vi "添加数据到配置文件.vi"(7 "参数GPRS引用句柄":refnum<vi>, 8 "错误输入（无错误）":errorcluster, 9 "配置文件输入":T1 caption="refnum", 10 "名称":string, 11 "下拉框输入":refnum<vi>) -> (0 "错误输出":errorcluster, 3 "配置文件输出":T1 caption="refnum out")   [LabVIEW 2015]
uses:
  <vilib>/Utility/config.llb/Config Data RefNum.ctl
  <vilib>/Utility/config.llb/Write Key (String).vi
  <vilib>/Utility/config.llb/Write Key (U32).vi
  <vilib>/Utility/config.llb/NI_LVConfig.lvlib
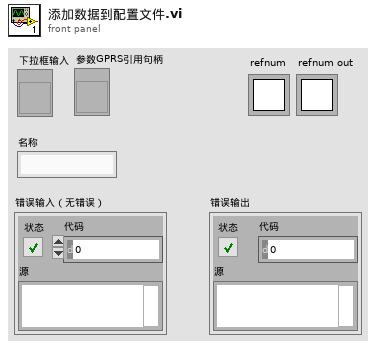
[diagram p1: front panel]
types:
  T1 = typedef "NI_LVConfig.lvlib/Config Data RefNum.ctl" = refnum<k1>
  T2 = typedef "GPRS参数123.ctl" = cluster{"IP地址":string, "端口号":u16, "工作模式":u16, "连接协议":u16, "连接方式":u16, "本机号码":string, "短信监控中心号码1":string, "监听时间":u16, "心跳间隔":u16, "重启时间(分)":u16, "C/S关系":u16, "DNS域名":string, "APN接入点":string, "报头使能":u16, "ID号":string, "波特率":u16, "数据位":u16, "停止位":u16, "校验位":u16, "短信目标号码1 ":string, "短信目标号码2":string, "短信监控中心号码2":string, "信号检测使能":u16, "控制方式":u16}
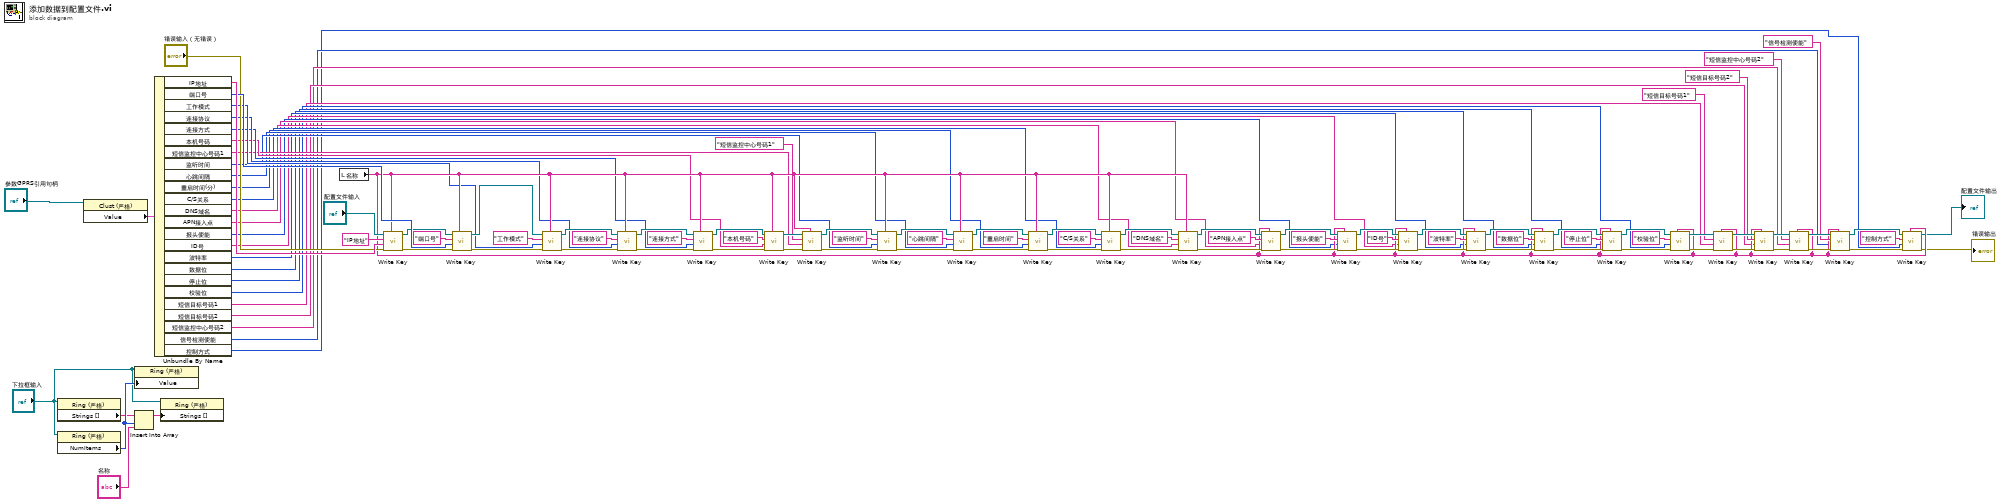
[diagram p0: block diagram]
diagram:
  n1 = property on="属性节点" class="Ring (严格)"(reference="下拉框输入") -> ("Strings []"=w105:string[])  [unwired: 1 in, 2 out]
  n2 = property on="属性节点" class="Ring (严格)"(reference="下拉框输入") -> ("NumItems"=w106:u32)  [unwired: 1 in, 2 out]
  n3 = property class="Clust (严格)"(reference="参数GPRS引用句柄") -> ("Value"=w101:T2)  [unwired: 1 in, 2 out]
  n4 = property on="属性节点" class="Ring (严格)"(reference="下拉框输入", "Value"=w106) -> ()  [unwired: 1 in, 2 out]
  n5 = Insert Into Array(array=w105, index=w106, new element="名称") -> (w104:string[])
  n6 = Unbundle By Name(w101) -> ("IP地址"=w98:string, "端口号"=w96:u16, "工作模式"=w24:u16, "连接协议"=w23:u16, "连接方式"=w22:u16, "本机号码"=w21:string, "短信监控中心号码1"=w20:string, "监听时间"=w19:u16, "心跳间隔"=w18:u16, "重启时间(分)"=w17:u16, "C/S关系"=w16:u16, "DNS域名"=w15:string, "APN接入点"=w14:string, "报头使能"=w13:u16, "ID号"=w12:string, "波特率"=w11:u16, "数据位"=w10:u16, "停止位"=w9:u16, "校验位"=w8:u16, "短信目标号码1"=w7:string, "短信目标号码2"=w6:string, "短信监控中心号码2"=w5:string, "信号检测使能"=w4:u16, "控制方式"=w3:u16)
  n7 = property on="属性节点" class="Ring (严格)"(reference="下拉框输入", "Strings []"=w104) -> ()  [unwired: 1 in, 2 out]
  n8 = local read "名称"() -> (w25:string)
  n9 = call-poly <vilib>:"Write Key.vi"("section"=w25, "error in (no error)"="错误输入（无错误）", "value"=w98, "key"="IP地址", "refnum"="配置文件输入") -> ("error out"=w92:errorcluster, "refnum out"=w94:T1)  [unwired: 4 in, 1 out]
  n10 = call-poly <vilib>:"Write Key.vi"("section"=w25, "error in (no error)"=w92, "value"=w96, "key"="端口号", "refnum"=w94) -> ("error out"=w60:errorcluster, "refnum out"=w61:T1)  [unwired: 4 in, 1 out]
  n11 = call-poly <vilib>:"Write Key.vi"("section"=w25, "error in (no error)"=w60, "value"=w24, "key"="工作模式", "refnum"=w61) -> ("error out"=w91:errorcluster, "refnum out"=w90:T1)  [unwired: 4 in, 1 out]
  n12 = call-poly <vilib>:"Write Key.vi"("section"=w25, "error in (no error)"=w91, "value"=w23, "key"="连接协议", "refnum"=w90) -> ("error out"=w87:errorcluster, "refnum out"=w86:T1)  [unwired: 4 in, 1 out]
  n13 = call-poly <vilib>:"Write Key.vi"("section"=w25, "error in (no error)"=w87, "value"=w22, "key"="连接方式", "refnum"=w86) -> ("error out"=w89:errorcluster, "refnum out"=w88:T1)  [unwired: 4 in, 1 out]
  n14 = call-poly <vilib>:"Write Key.vi"("section"=w25, "error in (no error)"=w89, "value"=w21, "key"="本机号码", "refnum"=w88) -> ("error out"=w79:errorcluster, "refnum out"=w78:T1)  [unwired: 4 in, 1 out]
  n15 = call-poly <vilib>:"Write Key.vi"("section"=w25, "error in (no error)"=w79, "value"=w20, "key"="短信监控中心号码1", "refnum"=w78) -> ("error out"=w85:errorcluster, "refnum out"=w84:T1)  [unwired: 4 in, 1 out]
  n16 = call-poly <vilib>:"Write Key.vi"("section"=w25, "error in (no error)"=w85, "value"=w19, "key"="监听时间", "refnum"=w84) -> ("error out"=w81:errorcluster, "refnum out"=w80:T1)  [unwired: 4 in, 1 out]
  n17 = call-poly <vilib>:"Write Key.vi"("section"=w25, "error in (no error)"=w81, "value"=w18, "key"="心跳间隔", "refnum"=w80) -> ("error out"=w83:errorcluster, "refnum out"=w82:T1)  [unwired: 4 in, 1 out]
  n18 = call-poly <vilib>:"Write Key.vi"("section"=w25, "error in (no error)"=w83, "value"=w17, "key"="重启时间", "refnum"=w82) -> ("error out"=w63:errorcluster, "refnum out"=w62:T1)  [unwired: 4 in, 1 out]
  n19 = call-poly <vilib>:"Write Key.vi"("section"=w25, "error in (no error)"=w63, "value"=w16, "key"="C/S关系", "refnum"=w62) -> ("error out"=w77:errorcluster, "refnum out"=w76:T1)  [unwired: 4 in, 1 out]
  n20 = call-poly <vilib>:"Write Key.vi"("section"=w25, "error in (no error)"=w77, "value"=w15, "key"="DNS域名", "refnum"=w76) -> ("error out"=w73:errorcluster, "refnum out"=w72:T1)  [unwired: 4 in, 1 out]
  n21 = call-poly <vilib>:"Write Key.vi"("section"=w25, "error in (no error)"=w73, "value"=w14, "key"="APN接入点", "refnum"=w72) -> ("error out"=w75:errorcluster, "refnum out"=w74:T1)  [unwired: 4 in, 1 out]
  n22 = call-poly <vilib>:"Write Key.vi"("section"=w25, "error in (no error)"=w75, "value"=w13, "key"="报头使能", "refnum"=w74) -> ("error out"=w65:errorcluster, "refnum out"=w64:T1)  [unwired: 4 in, 1 out]
  n23 = call-poly <vilib>:"Write Key.vi"("section"=w25, "error in (no error)"=w65, "value"=w12, "key"="ID号", "refnum"=w64) -> ("error out"=w71:errorcluster, "refnum out"=w70:T1)  [unwired: 4 in, 1 out]
  n24 = call-poly <vilib>:"Write Key.vi"("section"=w25, "error in (no error)"=w71, "value"=w11, "key"="波特率", "refnum"=w70) -> ("error out"=w67:errorcluster, "refnum out"=w66:T1)  [unwired: 4 in, 1 out]
  n25 = call-poly <vilib>:"Write Key.vi"("section"=w25, "error in (no error)"=w67, "value"=w10, "key"="数据位", "refnum"=w66) -> ("error out"=w69:errorcluster, "refnum out"=w68:T1)  [unwired: 4 in, 1 out]
  n26 = call-poly <vilib>:"Write Key.vi"("section"=w25, "error in (no error)"=w69, "value"=w9, "key"="停止位", "refnum"=w68) -> ("error out"=w30:errorcluster, "refnum out"=w31:T1)  [unwired: 4 in, 1 out]
  n27 = call-poly <vilib>:"Write Key.vi"("section"=w25, "error in (no error)"=w30, "value"=w8, "key"="校验位", "refnum"=w31) -> ("error out"=w41:errorcluster, "refnum out"=w40:T1)  [unwired: 4 in, 1 out]
  n28 = call-poly <vilib>:"Write Key.vi"("section"=w25, "error in (no error)"=w41, "value"=w7, "key"="短信目标号码1", "refnum"=w40) -> ("error out"=w43:errorcluster, "refnum out"=w42:T1)  [unwired: 4 in, 1 out]
  n29 = call-poly <vilib>:"Write Key.vi"("section"=w25, "error in (no error)"=w43, "value"=w6, "key"="短信目标号码2", "refnum"=w42) -> ("error out"=w28:errorcluster, "refnum out"=w27:T1)  [unwired: 4 in, 1 out]
  n30 = call-poly <vilib>:"Write Key.vi"("section"=w25, "error in (no error)"=w28, "value"=w5, "key"="短信监控中心号码2", "refnum"=w27) -> ("error out"=w35:errorcluster, "refnum out"=w34:T1)  [unwired: 4 in, 1 out]
  n31 = call-poly <vilib>:"Write Key.vi"("section"=w25, "error in (no error)"=w35, "value"=w4, "key"="信号检测使能", "refnum"=w34) -> ("error out"=w37:errorcluster, "refnum out"=w36:T1)  [unwired: 4 in, 1 out]
  n32 = call-poly <vilib>:"Write Key.vi"("section"=w25, "error in (no error)"=w37, "value"=w3, "key"="控制方式", "refnum"=w36) -> ("error out"=→"错误输出":errorcluster, "refnum out"=→"配置文件输出":T1)  [unwired: 4 in, 1 out]
